vi "Get Backup Folder Directory.vi"() -> (0 "Backup Folder Directory":path)   [LabVIEW 2021, in "EDT File IO.lvlib"]
uses:
  EDT File IO.lvlib
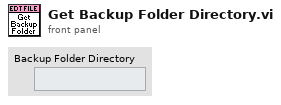
[diagram p1: front panel]
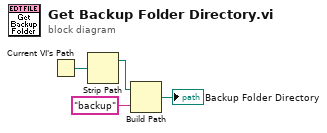
[diagram p0: block diagram]
diagram:
  n1 = Current VI's Path() -> (path=w1:path)
  n2 = Strip Path(path=w1) -> (stripped path=w2:path)  [unwired: 1 out]
  n3 = Build Path(base path=w2, name or relative path="backup" ("name")) -> (appended path=→"Backup Folder Directory":path)
